vi "Convert Arm Setting String to Parameters.vi"(6 "error in (no error)":errorcluster, 9 "Arm Mode Setting":string) -> (0 "error out":errorcluster, 3 "Angle":dbl, 4 "Enable Lock":bool)   [LabVIEW 2015]
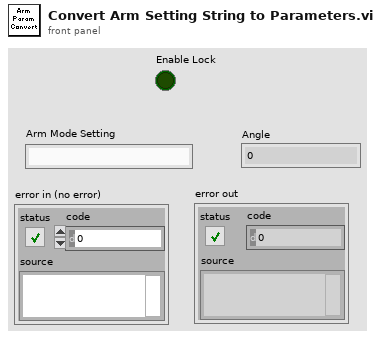
[diagram p1: front panel]
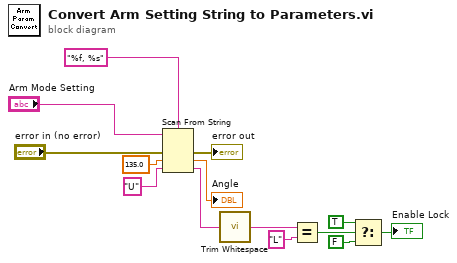
[diagram p0: block diagram]
diagram:
  n1 = Scan From String(format string="%f, %s", input string="Arm Mode Setting", error in="error in (no error)", default 1=135.0 ("default value 1"), default 2="U" ("default value 2")) -> (error out=→"error out":errorcluster, output 1=→"Angle":dbl, output 2=w11:string)  [unwired: 1 in, 2 out]
  n2 = call <vilib>:"Trim Whitespace.vi"("string"=w11) -> ("trimmed string"=w10:string)  [unwired: 1 in]
  n3 = Equal?(x=w10, y="L") -> (x = y?=w8:bool)
  n4 = Select(t=TRUE ("Enable Lock"), s=w8, f=FALSE) -> (s? t:f=→"Enable Lock":bool)
